vi "ReadMessageFile.vi"(8 "error in (no error)":errorcluster) -> (0 "error out":errorcluster, 3 "ServiceDefs":T1[](array[typedef]))   [LabVIEW 2017, in "MessageGen.lvlib"]
uses:
  <vilib>/addons/InsightCM/MessageBus/CodeGen/MessageGen.lvlib
  <vilib>/addons/InsightCM/MessageBus/CodeGen/controls/ServiceDef.ctl
  <vilib>/addons/InsightCM/MessageBus/CodeGen/controls/MessageDef.ctl
  <vilib>/addons/InsightCM/MessageBus/CodeGen/controls/ParameterDef.ctl
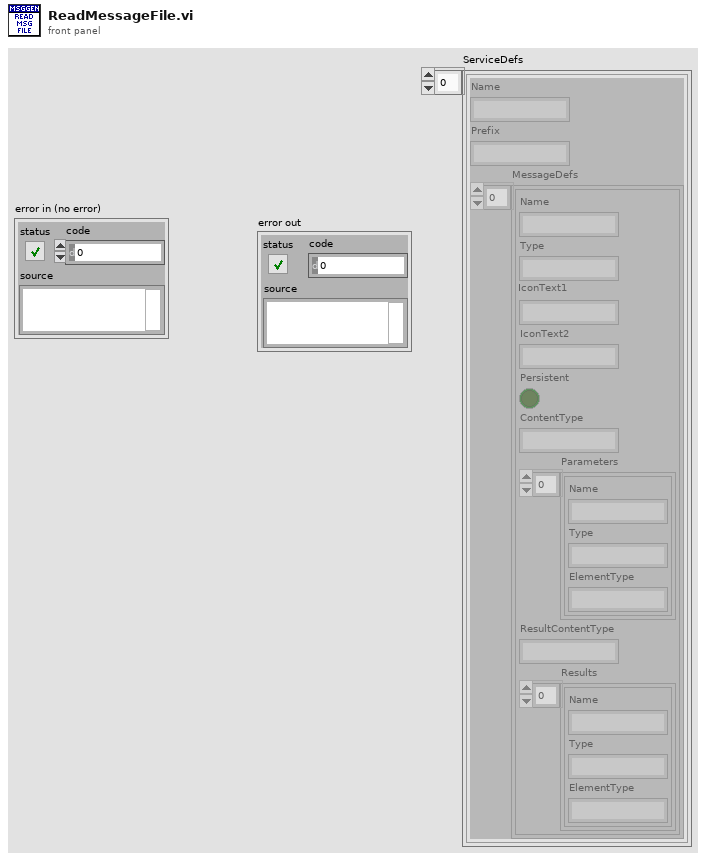
[diagram p1: front panel]
types:
  T1 = typedef "MessageGen.lvlib/ServiceDef.ctl" = cluster{"Name":string, "Prefix":string, "MessageDefs":T2[]}
  T2 = typedef "MessageGen.lvlib/MessageDef.ctl" = cluster{"Name":string, "Type":string, "IconText1":string, "IconText2":string, "Persistent":bool, "ContentType":string, "Parameters":T3[], "ResultContentType":string, "Results":T3[]}
  T3 = typedef "MessageGen.lvlib/ParameterDef.ctl" = cluster{"Name":string, "Type":string, "ElementType":string}
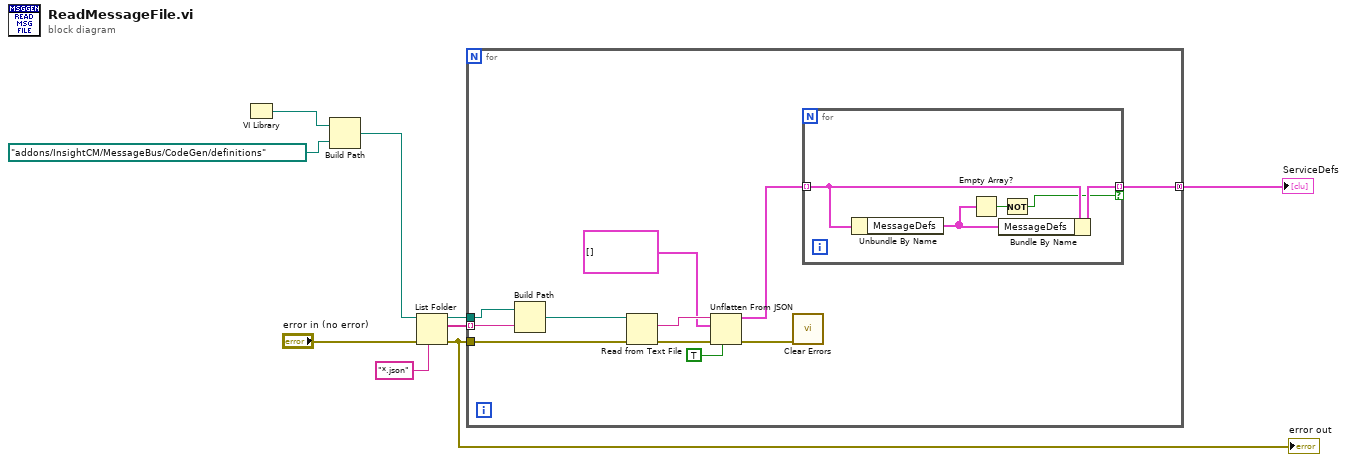
[diagram p0: block diagram]
diagram:
  n1 = VI Library() -> (path=w8:path)
  n2 = Build Path(base path=w8, name or relative path=path "addons/InsightCM/MessageBus/CodeGen/definitions") -> (appended path=w4:path)
  n3 = List Folder(path=w4, pattern="*.json", error in="error in (no error)") -> (path out=w3:path, filenames=w2:string[], error out=w1:errorcluster)  [unwired: 1 in, 1 out]
  "error out" <- w1
  n4 = for {
    tunnel: [w16] -> w9 mode=concatenating
    tunnel: w3 -> [w14]
    tunnel: w2 -> [w13] mode=indexing
    tunnel: w1 -> [w11]
    n5 = Build Path(base path=w14, name or relative path=w13) -> (appended path=w12:path)
    n6 = Read from Text File(file (use dialog)=w12, error in=w11) -> (text=w20:string, error out=w15:errorcluster)  [unwired: 2 in, 2 out]
    n7 = Unflatten From JSON(JSON string=w20, type and defaults=T1[] [] ("ServiceDefs"), default null elements? (F)=TRUE, error in (no error)=w15) -> (value=w17:T1[], error out=w10:errorcluster)  [unwired: 3 in]
    n8 = call <vilib>:"Clear Errors.vi"("error in (no error)"=w10) -> ()  [unwired: 5 in, 2 out]
    n9 = for {
      tunnel: w17 -> [w25] mode=indexing
      tunnel: [w24] -> w16 mode=indexing if=w22
      n10 = Unbundle By Name(w25) -> ("MessageDefs"=w21:T2[])
      n11 = Empty Array?(array=w21) -> (empty?=w23:bool)
      n12 = Bundle By Name(cluster=w25, "MessageDefs"=w21) -> (w24:T1)
      n13 = Not(x=w23) -> (.not. x?=w22:bool)
    }
  }
  "ServiceDefs" <- w9
